vi "3-5.vi"   [LabVIEW 2022 SP3]
types:
  T1 = enum16{"open", "replace", "create", "open or create", "replace or create", "replace or create with confirmation"}
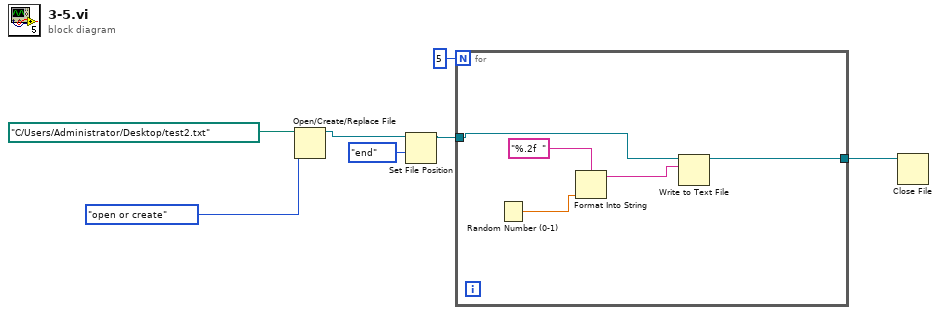
[diagram p0: block diagram]
diagram:
  n1 = Open/Create/Replace File(file path (use dialog)=path "C:/Users/Administrator/Desktop/test2.txt" ("文件路径（使用对话框）"), operation (0:open)=T1."open or create" ("操作(0:open)")) -> (refnum out=w5:refnum<file>)  [unwired: 4 in, 2 out]
  n2 = Set File Position(refnum=w5, from (0:start)=enum16{"start", "end", "current"}."end" ("自（0:起始）")) -> (refnum out=w2:refnum<file>)  [unwired: 2 in, 1 out]
  n3 = for {
    N: 5 -> [_]
    tunnel: w2 -> [w12]
    tunnel: [w8] -> w1
    n4 = Random Number (0-1)() -> (number: 0 to 1=w10:dbl)
    n5 = Format Into String(format string="%.2f  ", w10) -> (resulting string=w9:string)  [unwired: 2 in, 1 out]
    n6 = Write to Text File(file (use dialog)=w12, text=w9) -> (refnum out=w8:refnum<file>)  [unwired: 2 in, 2 out]
  }
  n7 = Close File(refnum=w1) -> ()  [unwired: 1 in, 2 out]
